vi "Get Table Name.vi"(8 "error in (no error)":errorcluster, 11 "Table Configuration in":refnum<class "Table Configuration.lvclass">) -> (0 "error out":errorcluster, 2 "Table Name":string, 3 "Table Configuration out":refnum<class "Table Configuration.lvclass">)   [LabVIEW 2020, in "Table.lvlib" / "Table Configuration.lvclass"]
uses:
  Table Configuration.lvclass
  Table Configuration.lvclass/Table Configuration.ctl
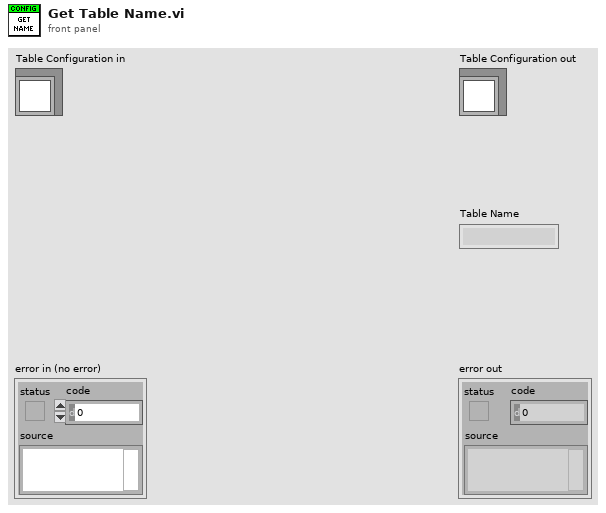
[diagram p1: front panel]
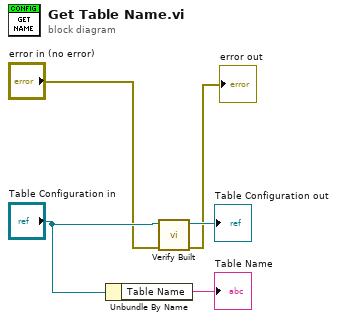
[diagram p0: block diagram]
diagram:
  n1 = Unbundle By Name("Table Configuration in") -> ("Table Name"=→"Table Name":string)
  n2 = call-dynamic "Verify Built.vi"("error in (no error)"="error in (no error)", "Table Configuration in"="Table Configuration in") -> ("error out"=→"error out":errorcluster, "Table Configuration out"=→"Table Configuration out":refnum<class "Table Configuration.lvclass">)  [unwired: 8 in]
